vi "Set IP Address.vi"(8 "error in (no error)":errorcluster, 10 "Value":string, 11 "Dev Ref in":T1 format="%.0x") -> (0 "error out":errorcluster, 3 "Dev Ref out":T1 format="%.0x")   [LabVIEW 2012, in "Image UDP Broadcast Custom Device.lvlib"]
uses:
  Image UDP Broadcast Custom Device.lvlib
  <vilib>/NI Veristand/Custom Device API/Custom Device Item Ref.ctl
  Image UDP Broadcast Global Variable.vi
  <vilib>/NI Veristand/Custom Device API/Set Item Property (String).vi
  <vilib>/NI Veristand/Custom Device API/Custom Device API.lvlib
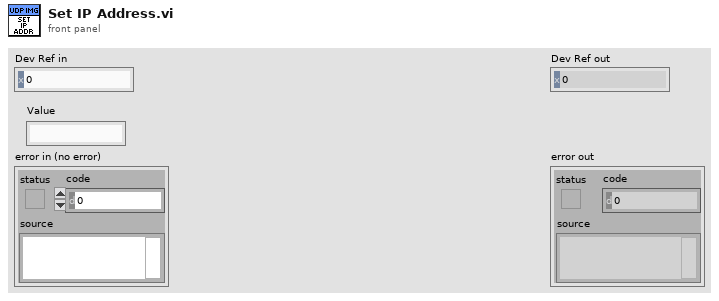
[diagram p1: front panel]
types:
  T1 = typedef "Custom Device API.lvlib/Custom Device Item Ref.ctl" = u64
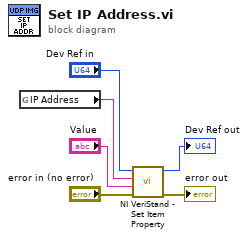
[diagram p0: block diagram]
diagram:
  n1 = global read "Image UDP Broadcast Global Variable.vi" "IP Address"() -> (w1:string)
  n2 = call-poly <vilib>:"NI VeriStand - Set Item Property.vi"("error in (no error)"="error in (no error)", "Value"="Value", "Property Name"=w1, "Item Ref in"="Dev Ref in") -> ("error out"=→"error out":errorcluster, "Item Ref out"=→"Dev Ref out":T1)  [unwired: 5 in, 1 out]
